vi "Progress_bar_subVI_BM.vi"(8 "Global Stop":bool, 10 "Current Iteration":i32, 11 "Runtime (min)":dbl) -> (0 "Loop Stop":bool, 3 "Progress Bar":u8(slide)=100 scale=0.0..100.0)   [LabVIEW 2021]
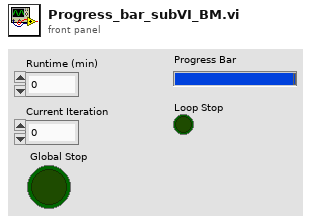
[diagram p1: front panel]
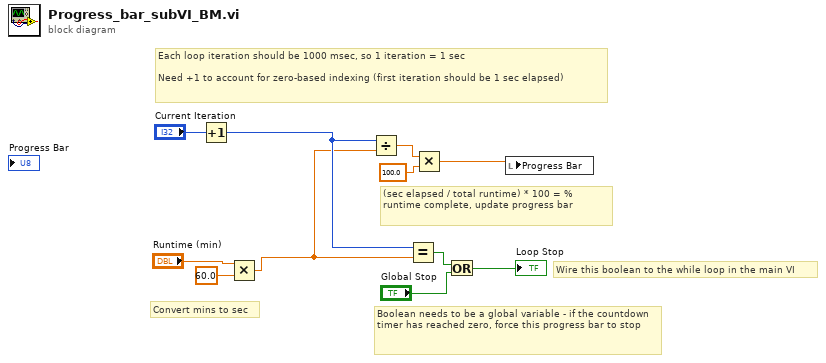
[diagram p0: block diagram]
diagram:
  # "Each loop iteration should be 1000 msec, so 1 iteration = 1 sec\n\nNeed +1 to account for zero-based indexing (first iteration should be 1 sec elapsed)"
  # "Wire this boolean to the while loop in the main VI"
  # "Boolean needs to be a global variable - if the countdown timer has reached zero, force this progress bar to stop"
  # "Convert mins to sec"
  # "(sec elapsed / total runtime) * 100 = % runtime complete, update progress bar"
  n1 = Increment(x="Current Iteration") -> (x+1=w8:i32)
  n2 = Multiply(x="Runtime (min)", y=60.0) -> (x*y=w2:dbl)
  n3 = Divide(x=w8, y=w2) -> (x/y=w6:dbl)
  n4 = Equal?(x=w8, y=w2) -> (x = y?=w9:bool)
  n5 = Multiply(x=w6, y=100.0) -> (x*y=w11:dbl)
  n6 = Or(x=w9, y="Global Stop") -> (x .or. y?=→"Loop Stop":bool)
  n7 = local write "Progress Bar"(w11) -> ()
